vi "arraybuilder.vi"(9 "Pin":string, 10 "ID":string, 11 "Name":string) -> (2 "Boolean":bool, 3 "Array":string[](array[string]))   [LabVIEW 2019]
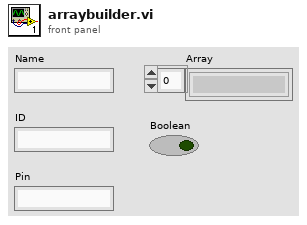
[diagram p1: front panel]
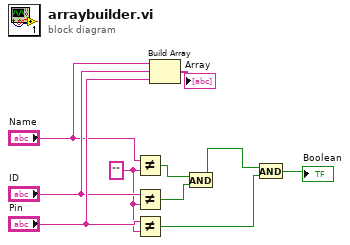
[diagram p0: block diagram]
diagram:
  w2 = "" ("y")
  n1 = Not Equal?(x="Name", y=w2) -> (x != y?=w3:bool)
  n2 = Not Equal?(x="ID", y=w2) -> (x != y?=w4:bool)
  n3 = Not Equal?(x="Pin", y=w2) -> (x != y?=w6:bool)
  n4 = Build Array("Name", "ID", "Pin") -> (→"Array":string[])
  n5 = And(x=w3, y=w4) -> (x .and. y?=w5:bool)
  n6 = And(x=w5, y=w6) -> (x .and. y?=→"Boolean":bool)
